vi "InjB-HMI.vi"() -> ()   [LabVIEW 2016]
uses:
  HV Controls.ctl
  Aperture RT Controls.ctl
  HV Readbacks.ctl
  Cryo Readbacks.ctl
  Bounce Field Readback.ctl
  Pressure Gauge.ctl
  Aperture RT Readbacks.ctl
  RT ctls.lvlib
panel:
  out "Injector Aperture Readbacks":T1
  out "Beam-line Pressure Gauge Readbacks":T2
  out "Ion Source Pressure Gauge Readbacks":T2
  out "Bounce Field Readbacks":T3
  out "Cryo Readbacks":T4
  in  "Bounce Magnet Set Value":dbl
  out "Injector HV Readbacks":T5
  in  "Injector Aperture Controls":T6
  in  "Injector HV Controls":T7
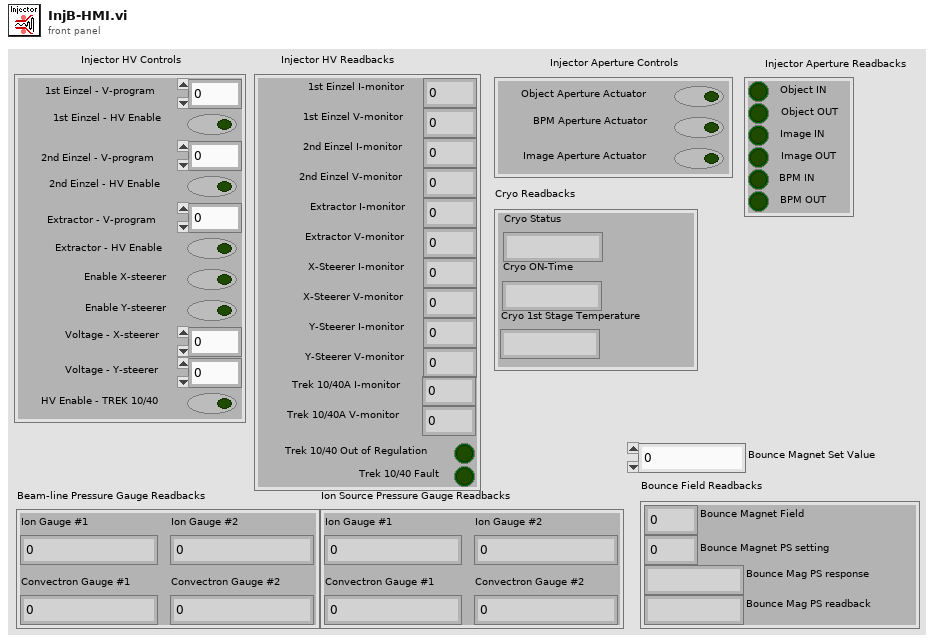
[diagram p1: front panel]
types:
  T1 = typedef "RT ctls.lvlib/Aperture RT Readbacks.ctl" = cluster{"Object IN":bool, "Object OUT":bool, "Image IN":bool, "Image OUT":bool, "BPM IN":bool, "BPM OUT":bool}
  T2 = typedef "RT ctls.lvlib/Pressure Gauge.ctl" = cluster{"Ion Gauge #1":dbl, "Convectron Gauge #1":dbl, "Convectron Gauge #2":dbl, "Ion Gauge #2":dbl}
  T3 = typedef "RT ctls.lvlib/Bounce Field Readback.ctl" = cluster{"Bounce Magnet Field":i32, "Bounce Mag PS response":string, "Bounce Mag PS readback":string, "Bounce Magnet PS setting":dbl}
  T4 = typedef "RT ctls.lvlib/Cryo Readbacks.ctl" = cluster{"Cryo Status":string, "Cryo ON-Time":string, "Cryo 1st Stage Temperature":string}
  T5 = typedef "RT ctls.lvlib/HV Readbacks.ctl" = cluster{"1st Einzel I-monitor":fxp<+/-,26,5>, "1st Einzel V-monitor":fxp<+/-,26,5>, "2nd Einzel I-monitor":fxp<+/-,26,5>, "2nd Einzel V-monitor":fxp<+/-,26,5>, "Extractor I-monitor":fxp<+/-,26,5>, "Extractor V-monitor":fxp<+/-,26,5>, "X-Steerer I-monitor":fxp<+/-,26,5>, "X-Steerer V-monitor":fxp<+/-,26,5>, "Y-Steerer I-monitor":fxp<+/-,26,5>, "Y-Steerer V-monitor":fxp<+/-,26,5>, "Trek 10/40 Out of Regulation":bool, "Trek 10/40 Fault":bool, "Trek 10/40A I-monitor":fxp<+/-,26,5>, "Trek 10/40A V-monitor":fxp<+/-,26,5>}
  T6 = typedef "RT ctls.lvlib/Aperture RT Controls.ctl" = cluster{"Object Aperture Actuator":bool, "BPM Aperture Actuator":bool, "Image Aperture Actuator":bool}
  T7 = typedef "RT ctls.lvlib/HV Controls.ctl" = cluster{"Enable X-steerer":bool, "Enable Y-steerer":bool, "Voltage - X-steerer":fxp<+/-,20,5>, "Voltage - Y-steerer":fxp<+/-,20,5>, "HV Enable - TREK 10/40":bool, "1st Einzel - V-program":fxp<+/-,20,5>, "1st Einzel - HV Enable":bool, "2nd Einzel - V-program":fxp<+/-,20,5>, "2nd Einzel - HV Enable":bool, "Extractor - V-program":fxp<+/-,20,5>, "Extractor - HV Enable":bool}
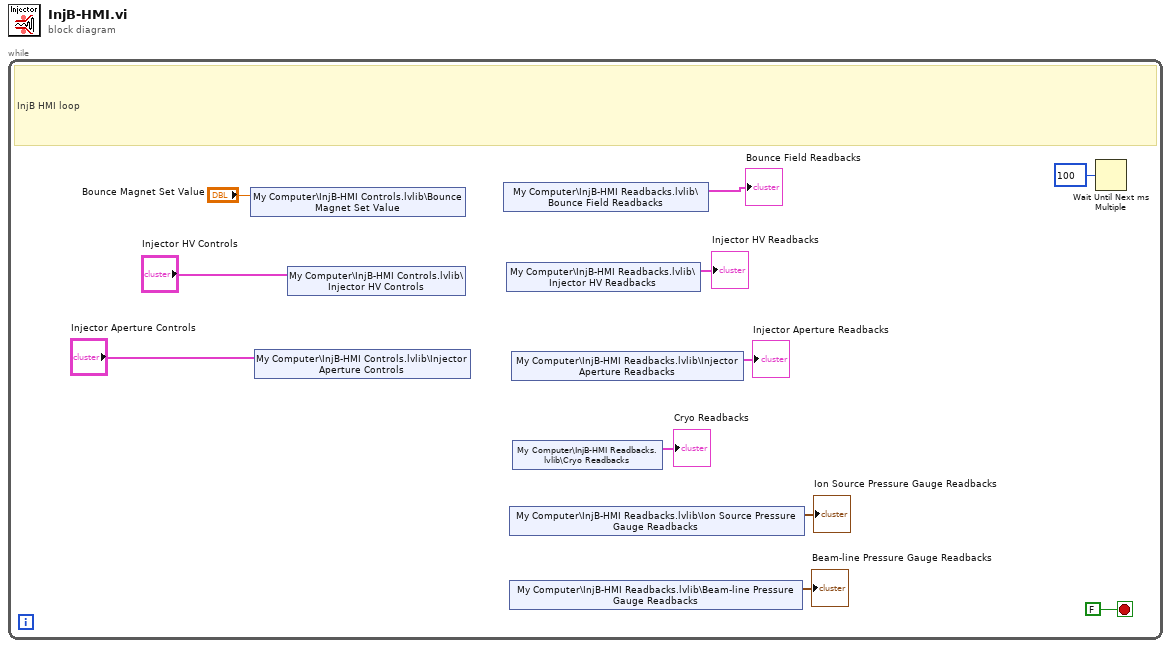
[diagram p0: block diagram]
diagram:
  n1 = while {
    stop <- FALSE stop-if-true
    # "InjB HMI loop"
    n2 = shared-variable "My Computer\\InjB-HMI Controls.lvlib\\Bounce Magnet Set Value"("Bounce Magnet Set Value") -> ()  [unwired: 1 in, 1 out]
    n3 = shared-variable "My Computer\\InjB-HMI Controls.lvlib\\Injector Aperture Controls"("Injector Aperture Controls") -> ()  [unwired: 1 in, 1 out]
    n4 = shared-variable "My Computer\\InjB-HMI Controls.lvlib\\Injector HV Controls"("Injector HV Controls") -> ()  [unwired: 1 in, 1 out]
    n5 = shared-variable "My Computer\\InjB-HMI Readbacks.lvlib\\Bounce Field Readbacks"() -> (→"Bounce Field Readbacks":T3)  [unwired: 1 in, 1 out]
    n6 = shared-variable "My Computer\\InjB-HMI Readbacks.lvlib\\Injector HV Readbacks"() -> (→"Injector HV Readbacks":T5)  [unwired: 1 in, 1 out]
    n7 = shared-variable "My Computer\\InjB-HMI Readbacks.lvlib\\Ion Source Pressure Gauge Readbacks"() -> (→"Ion Source Pressure Gauge Readbacks":T2)  [unwired: 1 in, 1 out]
    n8 = shared-variable "My Computer\\InjB-HMI Readbacks.lvlib\\Beam-line Pressure Gauge Readbacks"() -> (→"Beam-line Pressure Gauge Readbacks":T2)  [unwired: 1 in, 1 out]
    n9 = shared-variable "My Computer\\InjB-HMI Readbacks.lvlib\\Injector Aperture Readbacks"() -> (→"Injector Aperture Readbacks":T1)  [unwired: 1 in, 1 out]
    n10 = shared-variable "My Computer\\InjB-HMI Readbacks.lvlib\\Cryo Readbacks"() -> (→"Cryo Readbacks":T4)  [unwired: 1 in, 1 out]
    n11 = Wait Until Next ms Multiple(millisecond multiple=u32 100) -> ()  [unwired: 1 out]
  }
